vi "Actor Core.vi"(8 "error in":errorcluster, 11 "TopLevelApplication In":refnum<class "ConcreteViewModel.lvclass">) -> (0 "error out":errorcluster, 3 "Actor out":refnum<class "Actor.lvclass">)   [LabVIEW 2015, in "TopLevelApplication.lvlib" / "ConcreteViewModel.lvclass"]
doc: "(<B>Filename</B>: Actor Framework.lvlib:Actor.lvclass:Actor Core.vi)\n\nReceives messages to the actor, reacts to them, and initiates any error handling that may shut the actor down.\n\nDescendant classes may override this VI to append parallel tasks for the actor to complete while it handles messages. Overrides use the Call Parent Method node."
uses:
  ConcreteViewModel.lvclass
  <vilib>/ActorFramework/Actor/Actor.lvclass
  <vilib>/ActorFramework/Actor/Actor.lvclass/Actor.ctl
  <vilib>/ActorFramework/Message Enqueuer/Message Enqueuer.lvclass/Message Enqueuer.ctl
  <vilib>/ActorFramework/Message Enqueuer/Init from Existing Queue.vi
  <vilib>/ActorFramework/Message Enqueuer/Enqueue.vi
  <vilib>/ActorFramework/Message Priority Queue/Priority Enqueue.vi
  <vilib>/ActorFramework/Message Enqueuer/Message Enqueuer.lvclass
  <vilib>/ActorFramework/Stop Msg/Stop Msg.lvclass
  Framework/IViewModel/IViewModel/IViewModel.lvclass
panel:
  # "User-defined concrete Model Actor -- All UI stuff happens in the main subpanel\n(over this comment)"
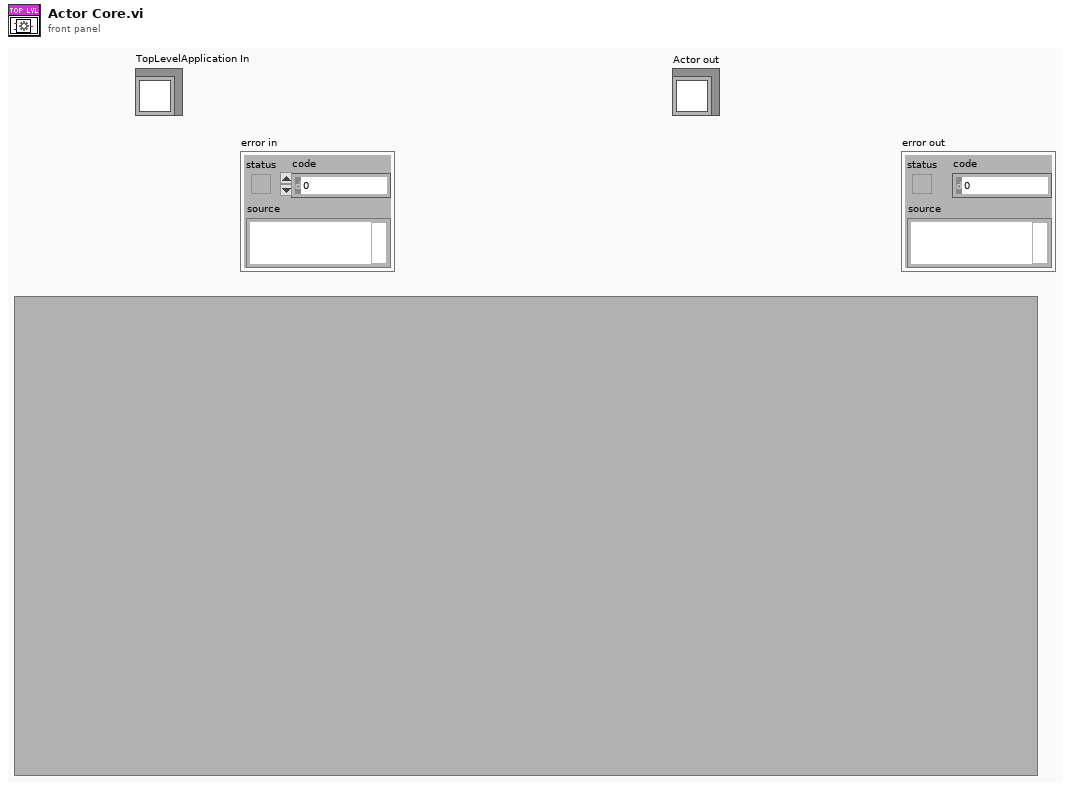
[diagram p1: front panel]
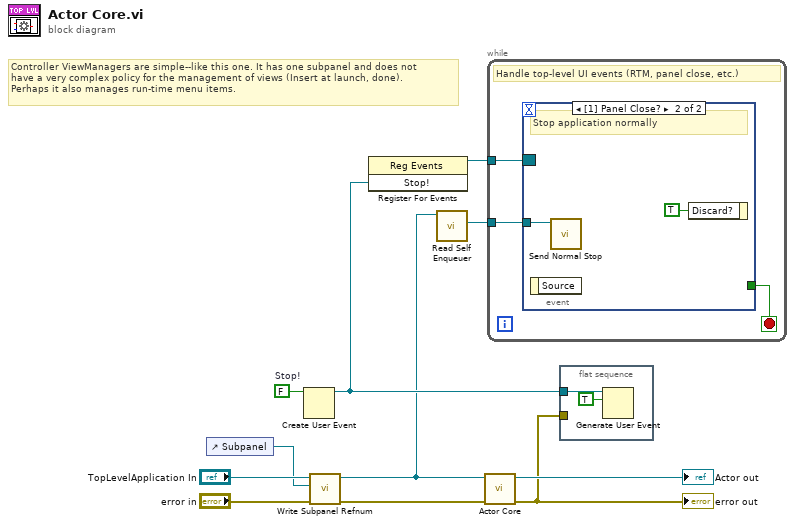
[diagram p0: block diagram]
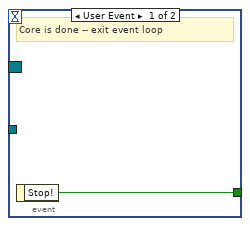
[diagram p2: hidden frame]
diagram:
  w10 = FALSE  # Stop!
  # "Controller ViewManagers are simple--like this one. It has one subpanel and does not\nhave a very complex policy for the management of views (Insert at launch, done).\nPerhaps it also manages run-time menu items."
  n1 = control-ref of="Subpanel"() -> (w1:refnum<vi>)
  n2 = Create User Event(user event datatype=w10) -> (user event=w8:refnum<user-event>)  [unwired: 1 in, 1 out]
  n3 = call "Write Subpanel Refnum.vi"("error in (no error)"="error in", "SubPnl Refnum"=w1, "IViewModel In"="TopLevelApplication In") -> ("error out"=w2:errorcluster, "IViewModel Out"=w4:refnum<class "ConcreteViewModel.lvclass">)  [unwired: 7 in]
  n4 = register-events(w8) -> (reference out=w9:refnum<event-registration>)  [unwired: 2 in, 1 out]
  n5 = call <vilib>:"Read Self Enqueuer.vi"("Actor"=w4) -> ("Self Enqueuer"=w6:refnum<class "Message Enqueuer.lvclass">)  [unwired: 10 in]
  n6 = call-parent "Actor Core.vi"("error in"=w2, "IViewModel In"=w4) -> ("error out"=w7:errorcluster, "Actor out"=→"Actor out":refnum<class "Actor.lvclass">)  [unwired: 8 in]
  "error out" <- w7
  n7 = while {
    tunnel: w9 -> [w14]
    tunnel: w6 -> [w12]
    stop <- w13 stop-if-true
    # "Handle top-level UI events (RTM, panel close, etc.)"
    n8 = event shown="[1] Panel Close?" {
      selector: w14 -> [_ _]
      dyn-events: _ -> [_ _]
      timeout: _ -> [_ _]
      tunnel: [w15 _] -> w13
      tunnel: w12 -> [_ w16]
      event User Event {
        # "Core is done -- exit event loop"
        n9 = event-data() -> ("Stop!"=w15:bool)  [unwired: 1 in]
      }
      event Panel Close? {
        # "Stop application normally"
        n10 = event-data() -> ()  [unwired: 1 in, 1 out]
        n11 = call <vilib>:"Send Normal Stop.vi"("Message Enqueuer"=w16) -> ()  [unwired: 10 in, 1 out]
        n12 = event-data("Discard?"=TRUE) -> ()  [unwired: 1 in, 1 out]
      }
    }
  }
  n13 = flat-sequence {
    tunnel: w8 -> [w19]
    tunnel: w7 -> [_]
    frame #0 {
      n14 = Generate User Event(user event=w19, event data cluster=TRUE ("event data")) -> ()  [unwired: 2 in, 2 out]
    }
  }
